vi "FXP32 TO I16 ARRRAY.vi"(0 "FXP32in":sgl, 1 "位数(2)":i32=2) -> (2 "L16":i16 format="%04x", 3 "H16":i16 format="%04x", 4 "out I16 array":i16[](array[numeric]) format="%04x")   [LabVIEW 2018]
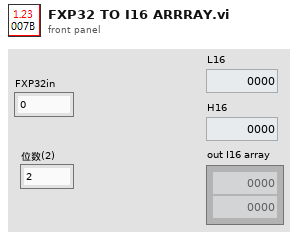
[diagram p1: front panel]
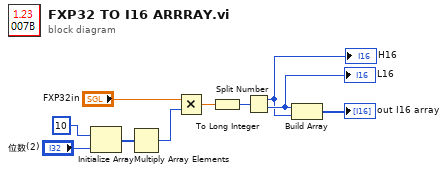
[diagram p0: block diagram]
diagram:
  n1 = Initialize Array(10 ("y"), "位数(2)") -> (w4:i32[])
  n2 = Multiply Array Elements(1:w4) -> (0:w3:i32)
  n3 = Multiply(x="FXP32in", y=w3) -> (x*y=w9:sgl)
  n4 = To Long Integer(number=w9) -> (32bit integer=w8:i32)
  n5 = Split Number(x=w8) -> (hi(x)=w1:u16, lo(x)=w2:u16)
  "L16" <- w2
  "H16" <- w1
  n6 = Build Array(w2, w1) -> (→"out I16 array":u16[])
